vi "AlliGator Phasor Plot Image ROI Storage [PM].vi"   [LabVIEW 2021, in "AlliGator ROIs.lvlib"]
doc: "Handles single or multiple Phasor Plot image ROI(s) storage."
uses:
  AlliGator ROIs.lvlib
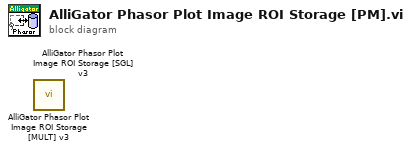
[diagram p0: block diagram]
diagram:
  n1 = call "AlliGator Phasor Plot Image ROI Storage [MULT] v3.vi"() -> ()  [unwired: 6 in, 6 out]
  n2 = call "AlliGator Phasor Plot Image ROI Storage [SGL] v3.vi"() -> ()  [unwired: 6 in, 6 out]
